vi "ScriptStringtoArray.vi"(1 "spreadsheet string":string) -> (0 "Array":string[](array[string]))   [LabVIEW 2016]
doc: "Converts a text file containing content and comments into an array of strings, with one array element for each row with content. All blank rows are also removed.\nCommented text is defined as all text following a \"#\" symbol on the same row."
uses:
  <vilib>/Utility/error.llb/whitespace.ctl
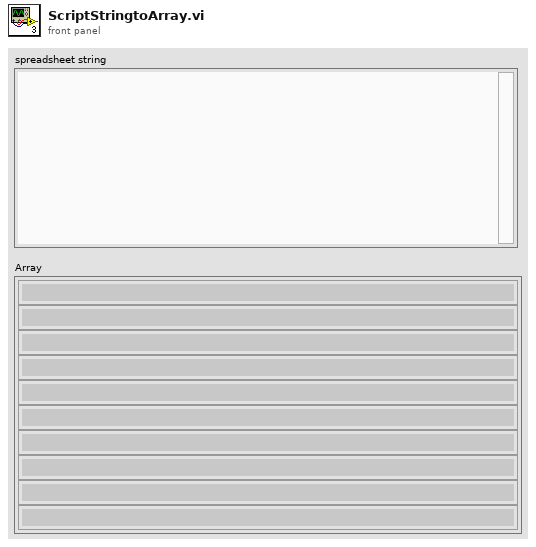
[diagram p1: front panel]
types:
  T1 = typedef "whitespace.ctl" = u16
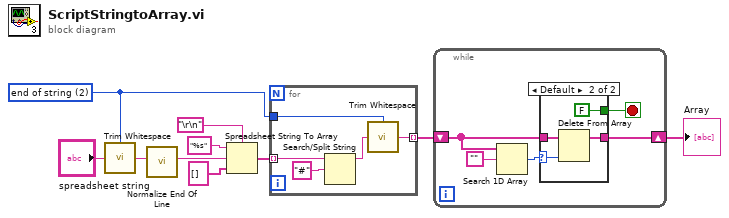
[diagram p0: block diagram]
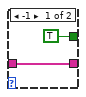
[diagram p2: hidden frame]
diagram:
  w2 = T1 2 items=["both", "start of string", "end of string"] ("location (both)")
  n1 = call <vilib>:"Trim Whitespace.vi"("string"="spreadsheet string", "location (both)"=w2) -> ("trimmed string"=w7:string)
  n2 = call <vilib>:"Normalize End Of Line.vi"("string in"=w7) -> ("string out"=w6:string)  [unwired: 7 in]
  n3 = Spreadsheet String To Array(delimiter (Tab)="\r\n", format string="%s", spreadsheet string=w6, array type (2D Dbl)=string[] []) -> (array=w5:string[])
  n4 = for {
    tunnel: w5 -> [w15] mode=indexing
    tunnel: [w12] -> w4 mode=indexing
    tunnel: w2 -> [w11]
    n5 = Search/Split String(string=w15, search string/char (-)="#") -> (substring before match=w13:string)  [unwired: 1 in, 2 out]
    n6 = call <vilib>:"Trim Whitespace.vi"("string"=w13, "location (both)"=w11) -> ("trimmed string"=w12:string)
  }
  n7 = while {
    shift-right: [w18] -> w3
    shift-left: w4 -> [w20]
    stop <- w19 stop-if-true
    n8 = Search 1D Array(1D array=w20, element="") -> (index of element=w17:i32)  [unwired: 1 in]
    n9 = case shown="Default" w17 {
      selector: w17 -> [_ w23]
      tunnel: w20 -> [w22 w26]
      tunnel: [w22 w25] -> w18
      tunnel: [TRUE FALSE] -> w19
      frame -1 {
      }
      frame Default {
        n10 = Delete From Array(array=w26, index=w23) -> (array with subset deleted=w25:string[])  [unwired: 1 in, 1 out]
      }
    }
  }
  "Array" <- w3
